vi "qudratic.vi"() -> ()   [LabVIEW 2024]
uses:
  <vilib>/Analysis/polynomials.llb/Polynomial Roots (DBL).vi
  <vilib>/Analysis/NI_AALPro.lvlib
panel:
  out "Roots":cdb[](array[numeric])
  out "x2":dbl
  out "x1":dbl
  in  "c":dbl
  in  "b":dbl
  in  "a":dbl
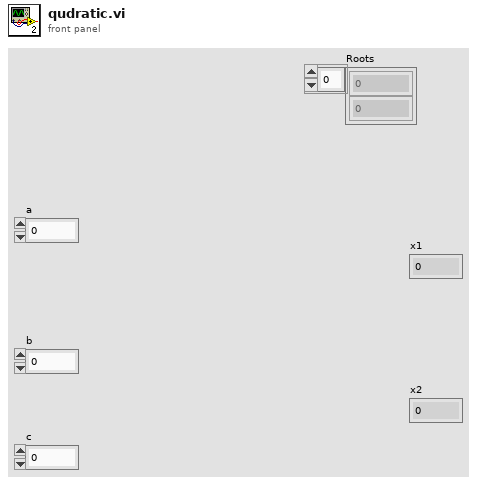
[diagram p1: front panel]
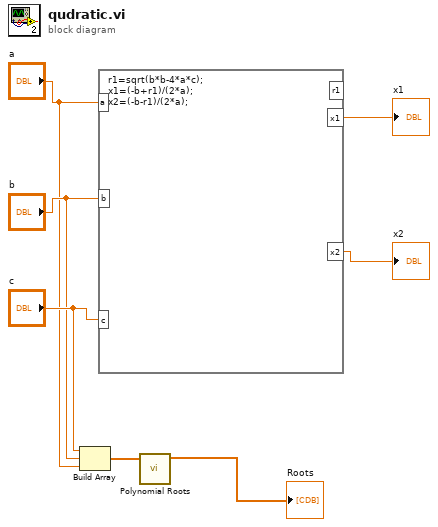
[diagram p0: block diagram]
diagram:
  n1 = Build Array("c", "b", "a") -> (w2:dbl[])
  n2 = formula code="r1=sqrt(b*b-4*a*c);\nx1=(-b+r1)/(2*a);\nx2=(-b-r1)/(2*a);"("b"="b", "a"="a", "c"="c") -> ("x1"=→"x1":dbl, "x2"=→"x2":dbl)  [unwired: 1 out]
  n3 = call-poly <vilib>:"Polynomial Roots.vi"("P(x)"=w2) -> ("Roots"=→"Roots":cdb[])  [unwired: 9 in, 1 out]
